vi "Pathhorafech_calibration.vi"(1 "Date Folder":string) -> (0 "path":path)   [LabVIEW 2015]
panel:
  out "date/time string":string
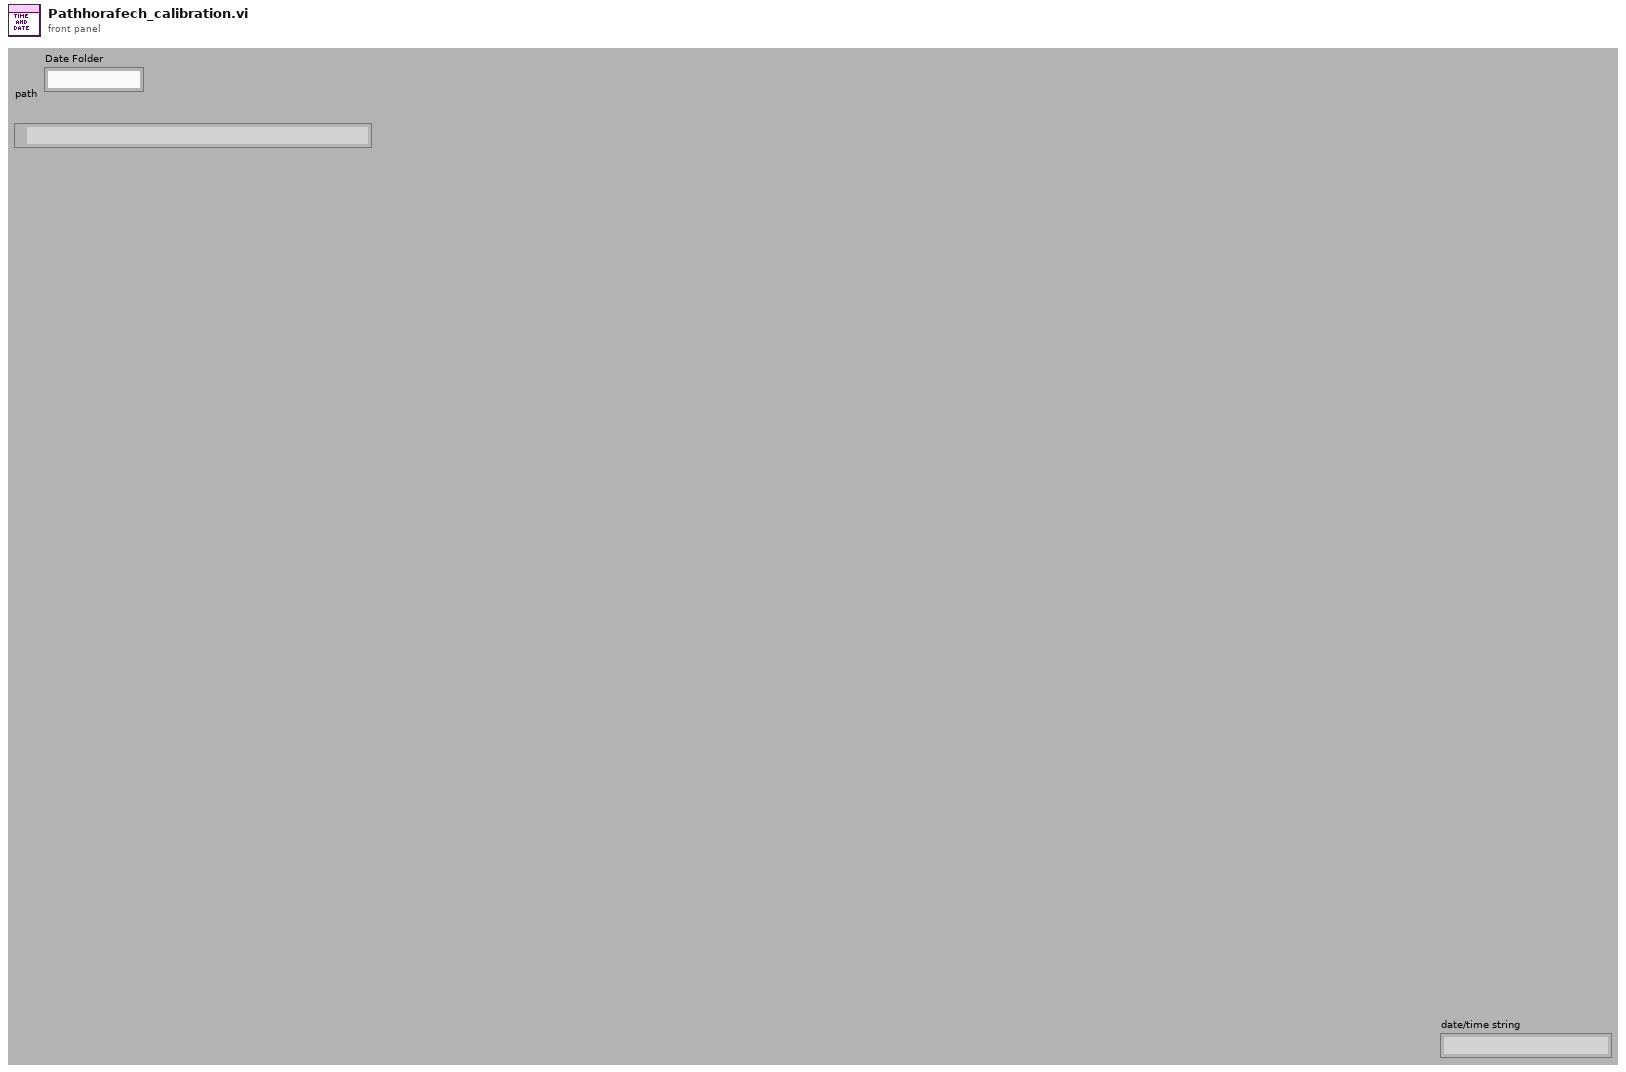
[diagram p1: front panel]
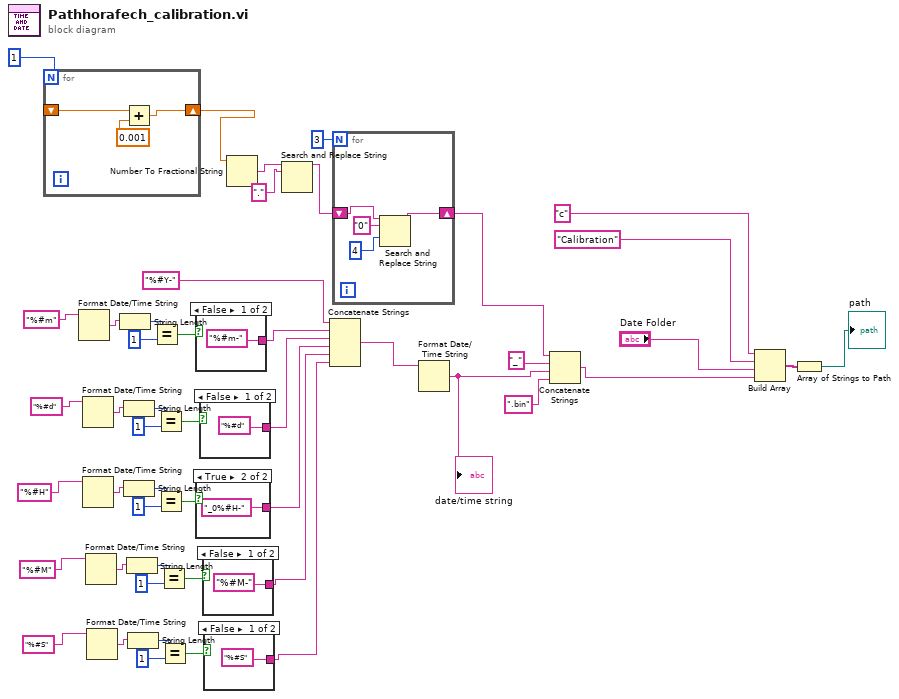
[diagram p0: block diagram]
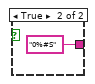
[diagram p2: hidden frame]
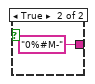
[diagram p3: hidden frame]
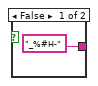
[diagram p4: hidden frame]
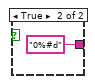
[diagram p5: hidden frame]
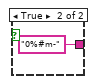
[diagram p6: hidden frame]
diagram:
  n1 = for {
    N: 1 -> [_]
    shift-right: [w51] -> w43
    shift-left: _ -> [w49]
    n2 = Add(x=w49, y=0.001) -> (x+y=w51:dbl)
  }
  n3 = Format Date/Time String(time format string (%c)="%#m") -> (date/time string=w30:string)  [unwired: 2 in]
  n4 = Format Date/Time String(time format string (%c)="%#d") -> (date/time string=w35:string)  [unwired: 2 in]
  n5 = Format Date/Time String(time format string (%c)="%#H") -> (date/time string=w19:string)  [unwired: 2 in]
  n6 = Format Date/Time String(time format string (%c)="%#M") -> (date/time string=w14:string)  [unwired: 2 in]
  n7 = Format Date/Time String(time format string (%c)="%#S") -> (date/time string=w9:string)  [unwired: 2 in]
  n8 = String Length(string=w30) -> (length=w31:i32)
  n9 = String Length(string=w35) -> (length=w36:i32)
  n10 = String Length(string=w19) -> (length=w20:i32)
  n11 = String Length(string=w14) -> (length=w15:i32)
  n12 = String Length(string=w9) -> (length=w10:i32)
  n13 = Equal?(x=w31, y=1) -> (x = y?=w33:bool)
  n14 = Equal?(x=w36, y=1) -> (x = y?=w38:bool)
  n15 = Equal?(x=w20, y=1) -> (x = y?=w22:bool)
  n16 = Equal?(x=w15, y=1) -> (x = y?=w17:bool)
  n17 = Equal?(x=w10, y=1) -> (x = y?=w12:bool)
  n18 = case shown="False" w33 {
    tunnel: ["%#m-" ("time format string (%c)") "0%#m-" ("time format string (%c)")] -> w40
    frame False {
    }
    frame True {
    }
  }
  n19 = case shown="True" w22 {
    tunnel: ["_%#H-" ("time format string (%c)") "_0%#H-" ("time format string (%c)")] -> w7
    frame False {
    }
    frame True {
    }
  }
  n20 = case shown="False" w38 {
    tunnel: ["%#d" ("time format string (%c)") "0%#d" ("time format string (%c)")] -> w41
    frame False {
    }
    frame True {
    }
  }
  n21 = case shown="False" w17 {
    tunnel: ["%#M-" ("time format string (%c)") "0%#M-" ("time format string (%c)")] -> w6
    frame False {
    }
    frame True {
    }
  }
  n22 = case shown="False" w12 {
    tunnel: ["%#S" ("time format string (%c)") "0%#S" ("time format string (%c)")] -> w5
    frame False {
    }
    frame True {
    }
  }
  n23 = Number To Fractional String(number=w43) -> (F-format string=w47:string)  [unwired: 3 out]
  n24 = Search and Replace String(input string=w47, search string="." ("replace string (\"\")")) -> (result string=w45:string)  [unwired: 1 in, 8 out]
  n25 = Concatenate Strings("%#Y-" ("time format string (%c)"), w40, w41, w7, w6, w5) -> (w42:string)
  n26 = for {
    N: 3 -> [_]
    shift-right: [w64] -> w4
    shift-left: w45 -> [w62]
    n27 = Search and Replace String(input string=w62, search string="0", offset=4 ("offset (0)")) -> (result string=w64:string)  [unwired: 1 in, 7 out]
  }
  n28 = Format Date/Time String(time format string (%c)=w42) -> (date/time string=w24:string)  [unwired: 2 in]
  "date/time string" <- w24
  n29 = Concatenate Strings(w4, "_" ("replace string (\"\")"), w24, ".bin" ("string")) -> (w28:string)
  n30 = Build Array("c", "Calibration" ("element"), "Date Folder", w28) -> (w27:string[])
  n31 = Array of Strings to Path(0:w27) -> (2:→"path":path)  [unwired: 1 out]
